vi "Remotely operated crane.vi"() -> ()   [LabVIEW 2024]
uses:
  <vilib>/MakerHub/PS4-Controller/Private/Type Defs/Indicators/Controller.ctl
  <vilib>/MakerHub/PS4-Controller/Private/Type Defs/Indicators/Square.ctl
  <vilib>/MakerHub/PS4-Controller/Private/Type Defs/Indicators/X.ctl
  <vilib>/MakerHub/PS4-Controller/Private/Type Defs/Indicators/Circle.ctl
  <vilib>/MakerHub/PS4-Controller/Private/Type Defs/Indicators/Triangle.ctl
  <vilib>/MakerHub/PS4-Controller/Private/Type Defs/Indicators/L1.ctl
  <vilib>/MakerHub/PS4-Controller/Private/Type Defs/Indicators/R1.ctl
  <vilib>/MakerHub/PS4-Controller/Private/Type Defs/Indicators/Share.ctl
  <vilib>/MakerHub/PS4-Controller/Private/Type Defs/Indicators/Options.ctl
  <vilib>/MakerHub/PS4-Controller/Private/Type Defs/Indicators/PS.ctl
  <vilib>/MakerHub/PS4-Controller/Private/Type Defs/Indicators/Pad_Button.ctl
  <vilib>/MakerHub/PS4-Controller/Private/Type Defs/Indicators/Dpad.ctl
  <vilib>/MakerHub/PS4-Controller/Private/Type Defs/Indicators/Slider.ctl
  <vilib>/MakerHub/PS4-Controller/Public/Open By Index.vi
  <vilib>/MakerHub/PS4-Controller/LMH-PS4.lvlib
panel:
  out "Numeric 2":u8
  out "Numeric":u8
  in  "Mode Select":bool
  in  "stop 2":bool
  out "Controller":T1={"Square Button"=FALSE, "X Button"=FALSE, "Circle Button"=FALSE, "Triangle Button"=FALSE, "L1"=FALSE, "R1"=FALSE, "Share Button"=FALSE, "Options Button"=FALSE, "PS Button"=FALSE, "Pad Button"=FALSE, "D-Pad"=5, "L2"=0, "R2"=0, "Thumbstick_Left"={[], []}, "Thumbstick_Right"={[], []}} {"R2" scale=-32768.0..32767.0; "L2" scale=-32768.0..32767.0}
  out "Servo 2":u8
  out "Servo 1":u8
  in  "IP address":string
  in  "Knob 2":u8(knob)=90 scale=65.0..135.0
  in  "Knob":u8(knob) scale=0.0..180.0
  in  "?":bool
  # "STOP servo"
  # "Max Wind in"
  # "Max Wind Out"
  # "CONTROLLER"
  # "HMI KNOBS"
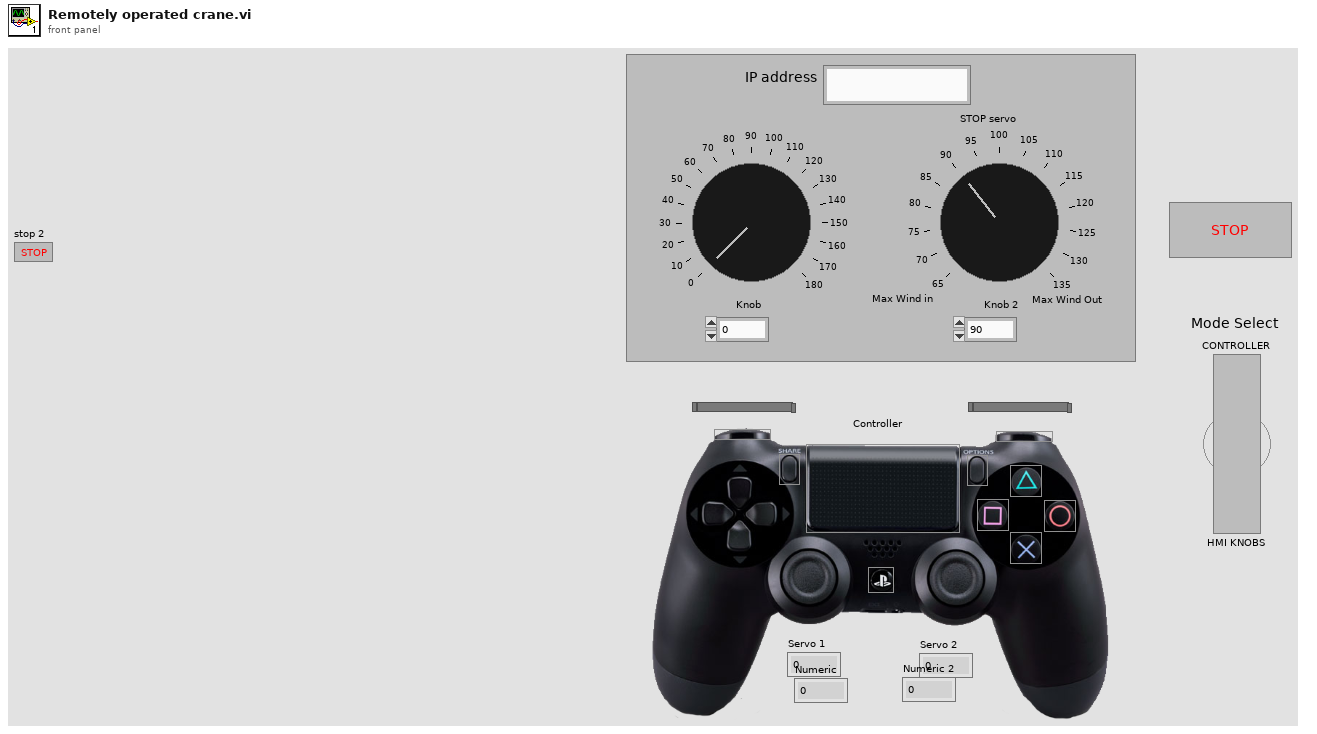
[diagram p1: front panel]
types:
  T1 = typedef "LMH-PS4.lvlib/Controller.ctl" = cluster{"Square Button":T2, "X Button":T3, "Circle Button":T4, "Triangle Button":T5, "L1":T6, "R1":T7, "Share Button":T8, "Options Button":T9, "PS Button":T10, "Pad Button":T11, "D-Pad":T12, "L2":T13, "R2":T13, "Thumbstick_Left":cluster{i32[], i32[]}, "Thumbstick_Right":cluster{i32[], i32[]}}
  T2 = typedef "LMH-PS4.lvlib/Square.ctl" = bool
  T3 = typedef "LMH-PS4.lvlib/X.ctl" = bool
  T4 = typedef "LMH-PS4.lvlib/Circle.ctl" = bool
  T5 = typedef "LMH-PS4.lvlib/Triangle.ctl" = bool
  T6 = typedef "LMH-PS4.lvlib/L1.ctl" = bool
  T7 = typedef "LMH-PS4.lvlib/R1.ctl" = bool
  T8 = typedef "LMH-PS4.lvlib/Share.ctl" = bool
  T9 = typedef "LMH-PS4.lvlib/Options.ctl" = bool
  T10 = typedef "LMH-PS4.lvlib/PS.ctl" = bool
  T11 = typedef "LMH-PS4.lvlib/Pad_Button.ctl" = bool
  T12 = typedef "LMH-PS4.lvlib/Dpad.ctl" = u16
  T13 = typedef "LMH-PS4.lvlib/Slider.ctl" = i32
  T14 = typedef "LMH-PS4.lvlib/PS4 Controller Ref.ctl" = cluster{"Controller Ref":refnum<k1>, "PS4 Events Ref":refnum<event-registration>, "Worker Ref":refnum<vi>}
  T15 = typedef "LMH-PS4.lvlib/Axis.ctl" = cluster{"Left Thumbstick":cluster{"X Axis":i32, "Y Axis":i32}, "Right Thumbstick":cluster{"X Axis":i32, "Y Axis":i32}, "L2":i32, "R2":i32, "D-Pad":T16}
  T16 = typedef "LMH-PS4.lvlib/DPad Enum.ctl" = enum16{"Idle", "Up", "Up / Right", "Right", "Down / Right", "Down", "Down / Left", "Left", "Up / Left"}
  T17 = typedef "LMH-PS4.lvlib/Buttons.ctl" = cluster{"Square":bool, "X":bool, "Circle":bool, "Triangle":bool, "L1":bool, "R1":bool, "L2":bool, "R2":bool, "Share":bool, "Options":bool, "Left Thumbstick":bool, "Right Thumbstick":bool, "Playstation Button":bool, "Pad":bool}
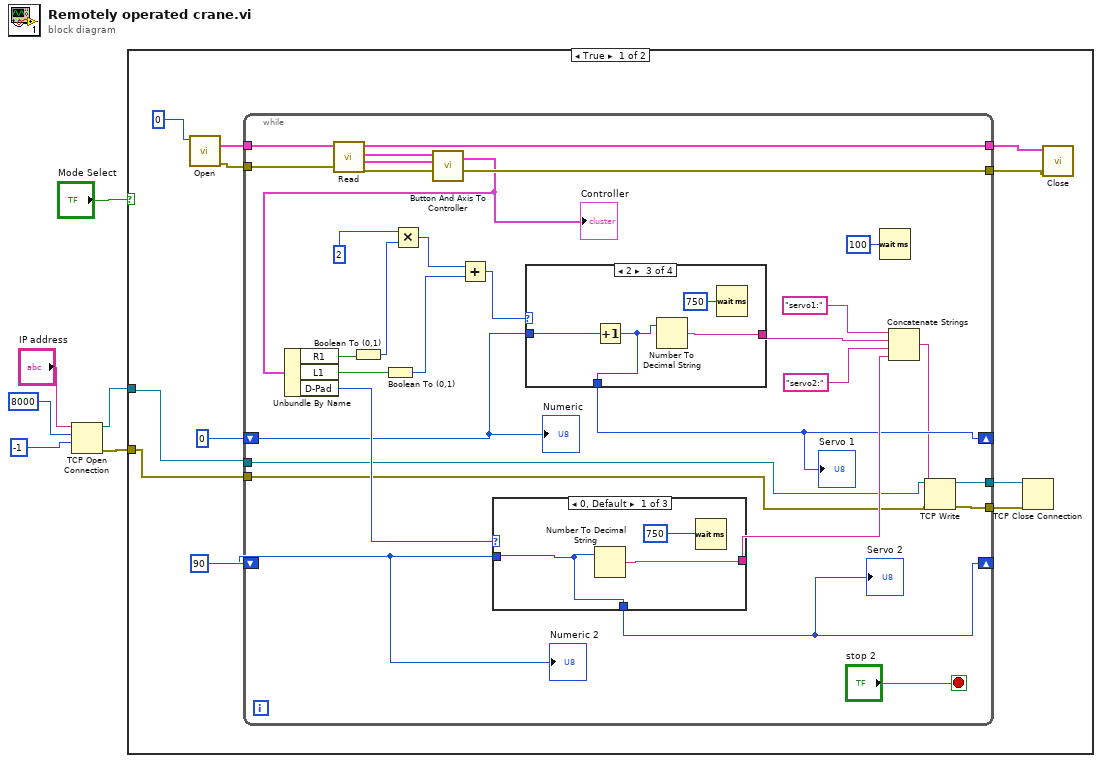
[diagram p0: block diagram]
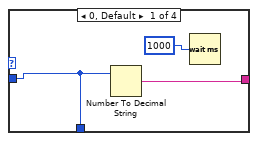
[diagram p2: hidden frame]
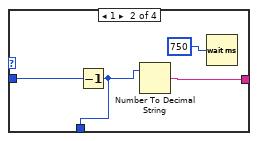
[diagram p3: hidden frame]
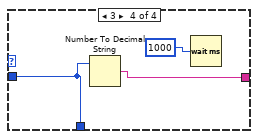
[diagram p4: hidden frame]
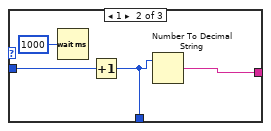
[diagram p5: hidden frame]
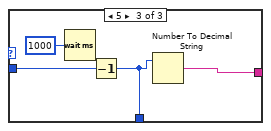
[diagram p6: hidden frame]
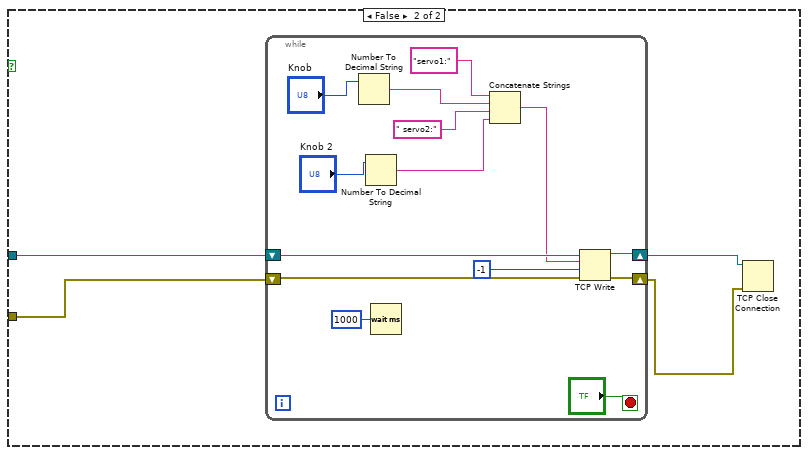
[diagram p7: hidden frame]
diagram:
  n1 = TCP Open Connection(address="IP address", remote port or service name=u16 8000, timeout ms (60000)=-1) -> (connection ID=w2:refnum<k5>, error out=w3:errorcluster)  [unwired: 2 in]
  n2 = case shown="True" "Mode Select" {
    tunnel: w3 -> [w9 w76]
    tunnel: w2 -> [w10 w75]
    frame True {
      n3 = call-poly <vilib>:"Open.vi"("Device Index"=0) -> ("Error Out"=w16:errorcluster, "PS4 Controller Ref"=w17:T14)  [unwired: 8 in, 1 out]
      n4 = while {
        tunnel: w17 -> [w46]
        tunnel: w16 -> [w45]
        tunnel: [w43] -> w15
        tunnel: [w42] -> w14
        shift-right: [w27] -> _
        shift-left: u8 0 -> [w18]
        shift-right: [w26] -> _
        shift-left: u8 90 -> [w19]
        tunnel: [w23] -> w7
        tunnel: [w22] -> w8
        tunnel: w10 -> [w21]
        tunnel: w9 -> [w20]
        stop <- "stop 2" stop-if-true
        n5 = call <vilib>:"Read.vi"("Error In"=w45, "PS4 Controller Ref"=w46) -> ("Error Out"=w42:errorcluster, "All Axis"=w44:T15, "Buttons"=w41:T17, "PS4 Controller Ref"=w43:T14)  [unwired: 6 in]
        n6 = call <vilib>:"Button And Axis To Controller.vi"("All Axis"=w44, "Buttons"=w41) -> ("PS4 Controller"=w40:T1)  [unwired: 5 in]
        "Controller" <- w40
        n7 = Unbundle By Name(w40) -> ("R1"=w36:T7, "L1"=w35:T6, "D-Pad"=w29:T12)
        n8 = Boolean To (0,1)(Boolean=w36) -> (0, 1=w32:i16)
        n9 = Boolean To (0,1)(Boolean=w35) -> (0, 1=w31:i16)
        n10 = Multiply(x=u16 2, y=w32) -> (x*y=w33:u16)
        n11 = Add(x=w33, y=w31) -> (x+y=w34:u16)
        n12 = case shown="0, Default" w29 {
          tunnel: w19 -> [w63 w68 w72]
          tunnel: [w64 w67 w71] -> w28
          tunnel: [w63 w66 w70] -> w26
          frame 0, Default {
            n13 = Number To Decimal String(number=w63) -> (decimal integer string=w64:string)  [unwired: 1 in]
            n14 = Wait (ms)(milliseconds to wait=u32 750) -> ()  [unwired: 1 out]
          }
          frame 1 {
            n15 = Wait (ms)(milliseconds to wait=u32 1000) -> ()  [unwired: 1 out]
            n16 = Increment(x=w68) -> (x+1=w66:u8)
            n17 = Number To Decimal String(number=w66) -> (decimal integer string=w67:string)  [unwired: 1 in]
          }
          frame 5 {
            n18 = Wait (ms)(milliseconds to wait=u32 1000) -> ()  [unwired: 1 out]
            n19 = Decrement(x=w72) -> (x-1=w70:u8)
            n20 = Number To Decimal String(number=w70) -> (decimal integer string=w71:string)  [unwired: 1 in]
          }
        }
        "Servo 2" <- w26
        n21 = case shown="2" w34 {
          tunnel: [w50 w54 w58 w61] -> w37
          tunnel: w18 -> [w49 w53 w57 w60]
          tunnel: [w49 w52 w56 w60] -> w27
          frame 0, Default {
            n22 = Number To Decimal String(number=w49) -> (decimal integer string=w50:string)  [unwired: 1 in]
            n23 = Wait (ms)(milliseconds to wait=u32 1000) -> ()  [unwired: 1 out]
          }
          frame 1 {
            n24 = Decrement(x=w53) -> (x-1=w52:u8)
            n25 = Number To Decimal String(number=w52) -> (decimal integer string=w54:string)  [unwired: 1 in]
            n26 = Wait (ms)(milliseconds to wait=u32 750) -> ()  [unwired: 1 out]
          }
          frame 2 {
            n27 = Increment(x=w57) -> (x+1=w56:u8)
            n28 = Number To Decimal String(number=w56) -> (decimal integer string=w58:string)  [unwired: 1 in]
            n29 = Wait (ms)(milliseconds to wait=u32 750) -> ()  [unwired: 1 out]
          }
          frame 3 {
            n30 = Number To Decimal String(number=w60) -> (decimal integer string=w61:string)  [unwired: 1 in]
            n31 = Wait (ms)(milliseconds to wait=u32 1000) -> ()  [unwired: 1 out]
          }
        }
        "Servo 1" <- w27
        n32 = Wait (ms)(milliseconds to wait=u32 100) -> ()  [unwired: 1 out]
        n33 = Concatenate Strings("servo1:" ("string"), w37, "servo2:" ("string"), w28) -> (w24:string)
        n34 = TCP Write(connection ID=w21, data in=w24, error in (no error)=w20) -> (connection ID out=w23:refnum<k5>, error out=w22:errorcluster)  [unwired: 1 in, 1 out]
        "Numeric" <- w18
        "Numeric 2" <- w19
      }
      n35 = TCP Close Connection(connection ID=w7, error in (no error)=w8) -> ()  [unwired: 1 in, 2 out]
      n36 = call <vilib>:"Close.vi"("Error In"=w14, "PS4 Controller Ref"=w15) -> ()  [unwired: 9 in, 1 out]
    }
    frame False {
      n37 = while {
        shift-right: [w89] -> w74
        shift-left: w75 -> [w85]
        shift-right: [w90] -> w73
        shift-left: w76 -> [w84]
        stop <- "?" stop-if-true
        n38 = Number To Decimal String(number="Knob") -> (decimal integer string=w81:string)  [unwired: 1 in]
        n39 = Number To Decimal String(number="Knob 2") -> (decimal integer string=w77:string)  [unwired: 1 in]
        n40 = Wait (ms)(milliseconds to wait=u32 1000) -> ()  [unwired: 1 out]
        n41 = Concatenate Strings("servo1:" ("string"), w81, " servo2:" ("string"), w77) -> (w79:string)
        n42 = TCP Write(connection ID=w85, data in=w79, error in (no error)=w84, 9:-1 ("timeout ms (25000)")) -> (connection ID out=w89:refnum<k5>, error out=w90:errorcluster)  [unwired: 1 out]
      }
      n43 = TCP Close Connection(connection ID=w74, error in (no error)=w73) -> ()  [unwired: 1 in, 2 out]
    }
  }
